vi "AndorSnap.vi"() -> ()   [LabVIEW 2014]
uses:
  <userlib>/atmcd64d.llb/AcquisitionMode_mode typedef.ctl
  <userlib>/atmcd64d.llb/ReadMode_mode typedef.ctl
  <userlib>/atmcd64d.llb/Shutter_mode typedef.ctl
  <userlib>/atmcd64d.llb/Shutter_type typedef.ctl
  <userlib>/atmcd64d.llb/TriggerMode_mode typedef.ctl
  <userlib>/atmcd64d.llb/Error Code Enum typedef.ctl
panel:
  out "SaveStatus":bool
  in  "FilePath":string="C:\\Users\\light\\Desktop\\Chuanzhen\\Andor\\data"
  out "ShutDown":cluster{"CoolOff":bool, "ShutDown":bool}
  in  "Set":bool
  in  "Snap":bool
  out "SetStatus":bool
  out "SetOut":T1
  out "Timing":T2 {"kinetic" format="%.2f"; "accumulate" format="%.2f"; "exposure" format="%.2f"}
  in  "MultiTrack":cluster{"StartRow":i32, "EndRow":i32}={"StartRow"=1, "EndRow"=256}
  in  "AcqSet":T3={"openingtime"=20, "closingtime"=20, "ExposureTime"=0.01, "AccumCycTime"=0.0, "AccumCycNum"=1, "KineticNum"=1, "KineticTime"=0.0} {"KineticTime" format="%.2f"; "AccumCycTime" format="%.2f"; "ExposureTime" format="%.2f"}
  in  "Mode":T9={"AcqMode"=enum."Single Scan", "ReadMode"=enum."Image", "ShutterMode"=enum."Auto", "GateMode"=enum."TTL High", "TriggerMode"=enum."Internal"}
  in  "Exit":bool
  out "CoolerON":T10
  out "CurrentTemp":i32
  out "GetStatus":T11
  out "Speeds":T12
  out "SoftWVersion":T13
  out "HardWVersion":T14
  out "DevSize":cluster{"xpixels":i32, "ypixels":i32}
  out "DevInit":bool
  in  "TargetTemp":i32
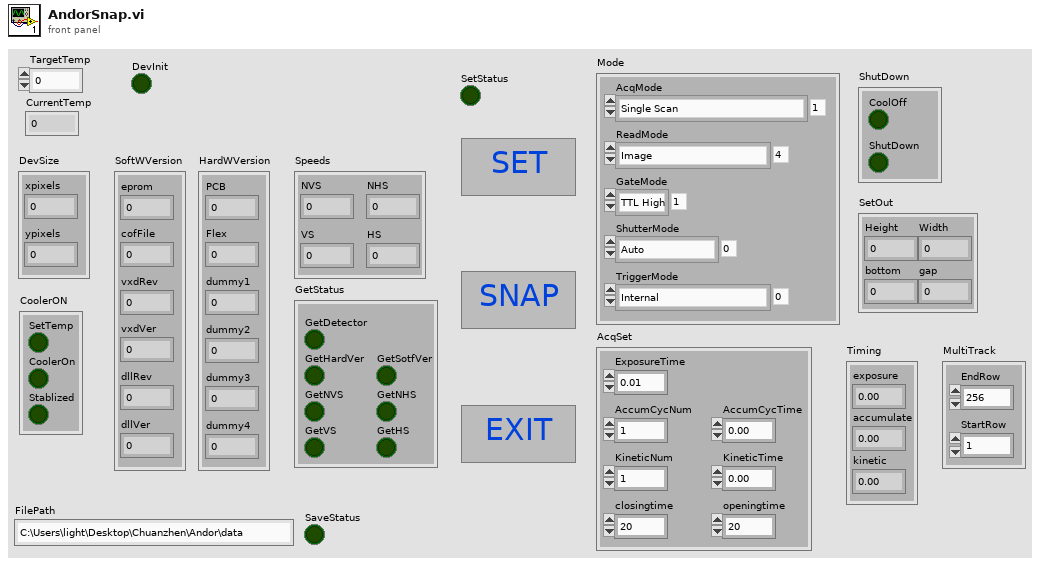
[diagram p1: front panel]
types:
  T1 = cluster{"Height":i32, "Width":i32, "bottom":i32, "gap":i32}
  T2 = cluster{"exposure":sgl, "accumulate":sgl, "kinetic":sgl}
  T3 = cluster{"openingtime":i32, "closingtime":i32, "ExposureTime":sgl, "AccumCycTime":sgl, "AccumCycNum":i32, "KineticNum":i32, "KineticTime":sgl}
  T4 = typedef "AcquisitionMode_mode typedef.ctl" = enum16{"Reserved (0)", "Single Scan", "Accumulate", "Kinetics", "Fast Kinetics", "Run Till Abort", "Reserved (6)", "Reserved (7)", "Reserved (8)", "Time Delayed Integration"}
  T5 = typedef "ReadMode_mode typedef.ctl" = enum16{"Full Vertical Binning", "Multi-Track", "Random-Track", "Single-Track", "Image"}
  T6 = typedef "Shutter_mode typedef.ctl" = enum16{"Auto", "Open", "Close", "N/A (3)", "Open FVB Series", "Open Any Series"}
  T7 = typedef "Shutter_type typedef.ctl" = enum16{"TTL Low", "TTL High"}
  T8 = typedef "TriggerMode_mode typedef.ctl" = enum16{"Internal", "External", "N/A (2)", "N/A (3)", "N/A (4)", "N/A (5)", "External Start", "External Exposure (Bulb)", "N/A (8)", "External FVB EM", "Software", "N/A (11)", "External Charge Shifting"}
  T9 = cluster{"AcqMode":T4, "ReadMode":T5, "ShutterMode":T6, "GateMode":T7, "TriggerMode":T8}
  T10 = cluster{"SetTemp":bool, "CoolerOn":bool, "Stablized":bool}
  T11 = cluster{"GetDetector":bool, "GetHardVer":bool, "GetNVS":bool, "GetVS":bool, "GetSotfVer":bool, "GetNHS":bool, "GetHS":bool}
  T12 = cluster{"NVS":i32, "VS":i32, "NHS":dbl, "HS":i32}
  T13 = cluster{"eprom":u32, "cofFile":u32, "vxdRev":u32, "vxdVer":u32, "dllRev":u32, "dllVer":u32}
  T14 = cluster{"PCB":u32, "Flex":u32, "dummy1":u32, "dummy2":u32, "dummy3":u32, "dummy4":u32}
  T15 = typedef "Error Code Enum typedef.ctl" = enum32{"N/A (0)", "DRV_ERROR_CODES", "DRV_SUCCESS", "DRV_VXDNOTINSTALLED", "DRV_ERROR_SCAN", "DRV_ERROR_CHECK_SUM", "DRV_ERROR_FILELOAD", "DRV_UNKNOWN_FUNC", "DRV_ERROR_VXD_INIT", "DRV_ERROR_ADDRESS", "DRV_ERROR_PAGELOCK", "DRV_ERROR_PAGEUNLOCK", "DRV_ERROR_BOARDTEST", "DRV_ERROR_ACK", "DRV_ERROR_UP_FIFO", "DRV_ERROR_PATTERN", "N/A (16)", "DRV_ACQUISITION_ERRORS", "DRV_ACQ_BUFFER", "DRV_ACQ_DOWNFIFO_FULL", "DRV_PROC_UNKONWN_INSTRUCTION", "DRV_ILLEGAL_OP_CODE", "DRV_KINETIC_TIME_NOT_MET", "DRV_ACCUM_TIME_NOT_MET", "DRV_NO_NEW_DATA", "N/A (25)", "DRV_SPOOLERROR", "N/A (27)", "N/A (28)", "N/A (29)", "N/A (30)", "N/A (31)", "N/A (32)", "DRV_TEMPERATURE_CODES", "DRV_TEMPERATURE_OFF", "DRV_TEMPERATURE_NOT_STABILIZED", "DRV_TEMPERATURE_STABILIZED", "DRV_TEMPERATURE_NOT_REACHED", "DRV_TEMPERATURE_OUT_RANGE", "DRV_TEMPERATURE_NOT_SUPPORTED", "DRV_TEMPERATURE_DRIFT", "N/A (41)", "N/A (42)", "N/A (43)", "N/A (44)", "N/A (45)", "N/A (46)", "N/A (47)", "N/A (48)", "DRV_GENERAL_ERRORS", "DRV_INVALID_AUX", "DRV_COF_NOTLOADED", "DRV_FPGAPROG", "DRV_FLEXERROR", "DRV_GPIBERROR", "N/A (55)", "N/A (56)", "N/A (57)", "N/A (58)", "N/A (59)", "N/A (60)", "N/A (61)", "N/A (62)", "N/A (63)", "DRV_DATATYPE", "DRV_DRIVER_ERRORS", "DRV_P1INVALID", "DRV_P2INVALID", "DRV_P3INVALID", "DRV_P4INVALID", "DRV_INIERROR", "DRV_COFERROR", "DRV_ACQUIRING", "DRV_IDLE", "DRV_TEMPCYCLE", "DRV_NOT_INITIALIZED", "DRV_P5INVALID", "DRV_P6INVALID", "DRV_INVALID_MODE", "DRV_INVALID_FILTER", "DRV_I2CERRORS", "DRV_I2CDEVNOTFOUND", "DRV_I2CTIMEOUT", "DRV_P7INVALID", "N/A (84)", "N/A (85)", "N/A (86)", "N/A (87)", "N/A (88)", "N/A (89)", "DRV_IOCERROR", "DRV_VRMVERSIONERROR"}
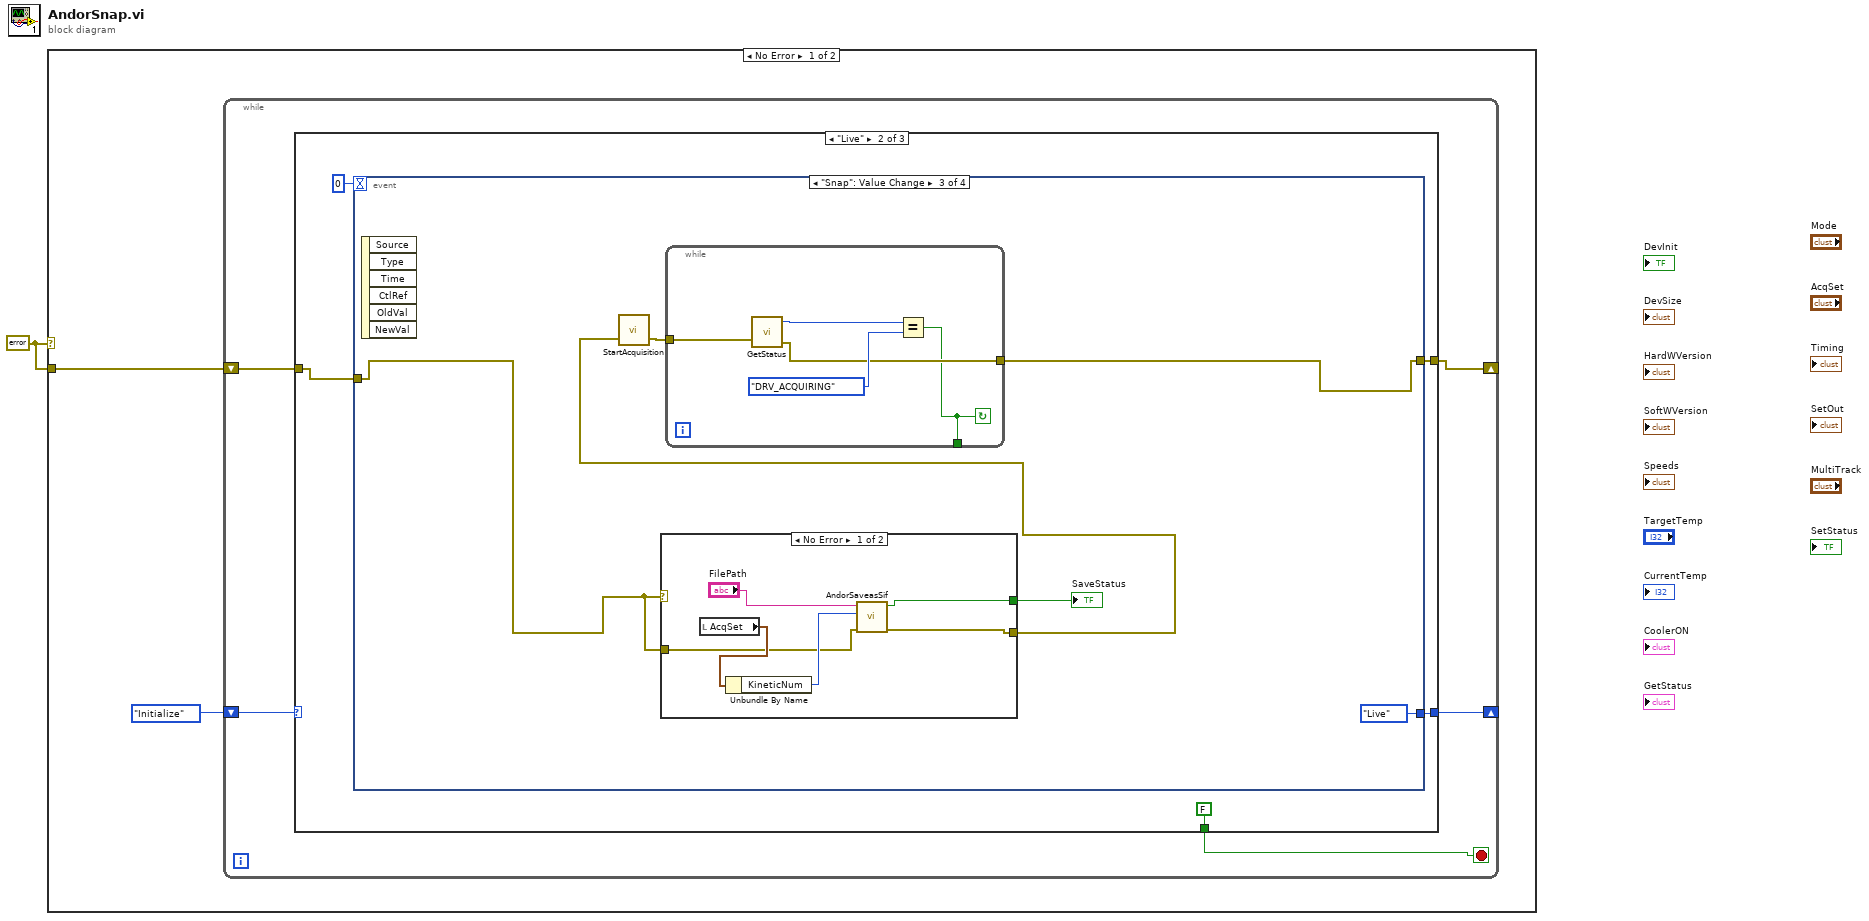
[diagram p0: block diagram]
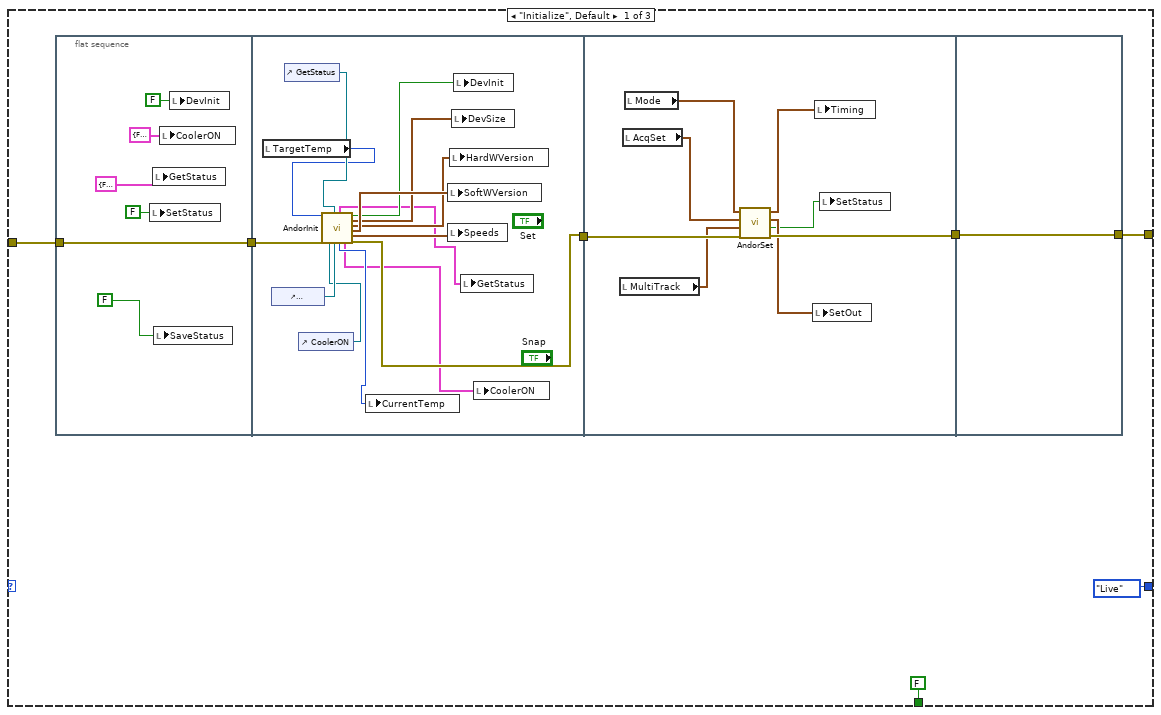
[diagram p2: hidden frame]
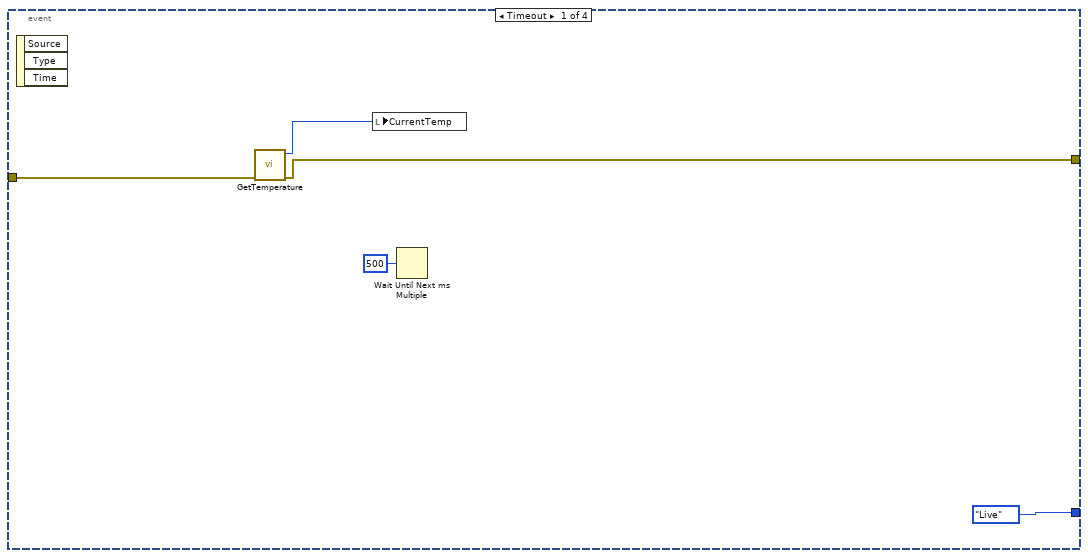
[diagram p3: hidden frame]
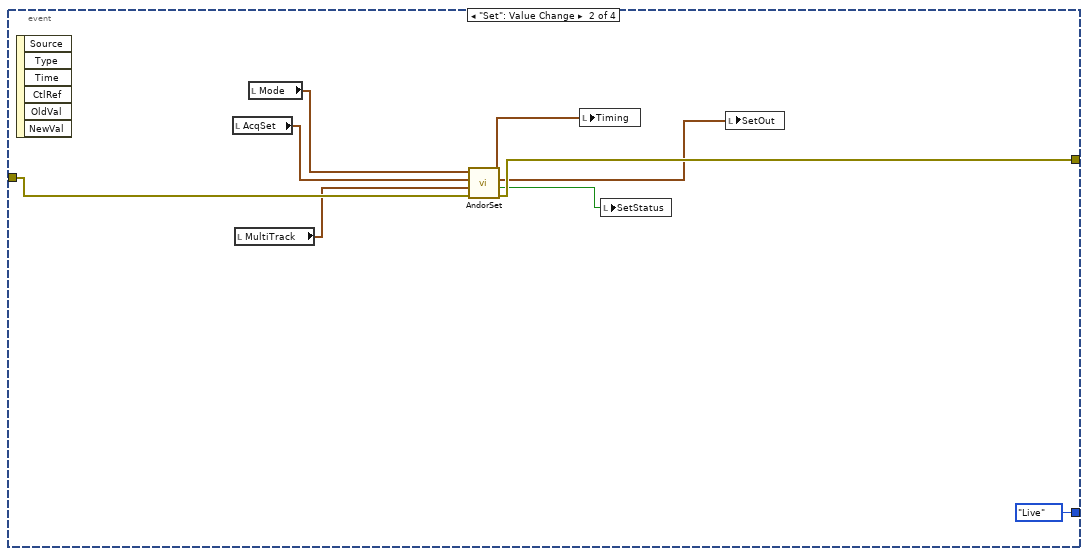
[diagram p4: hidden frame]
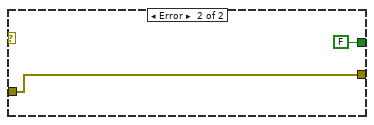
[diagram p5: hidden frame]
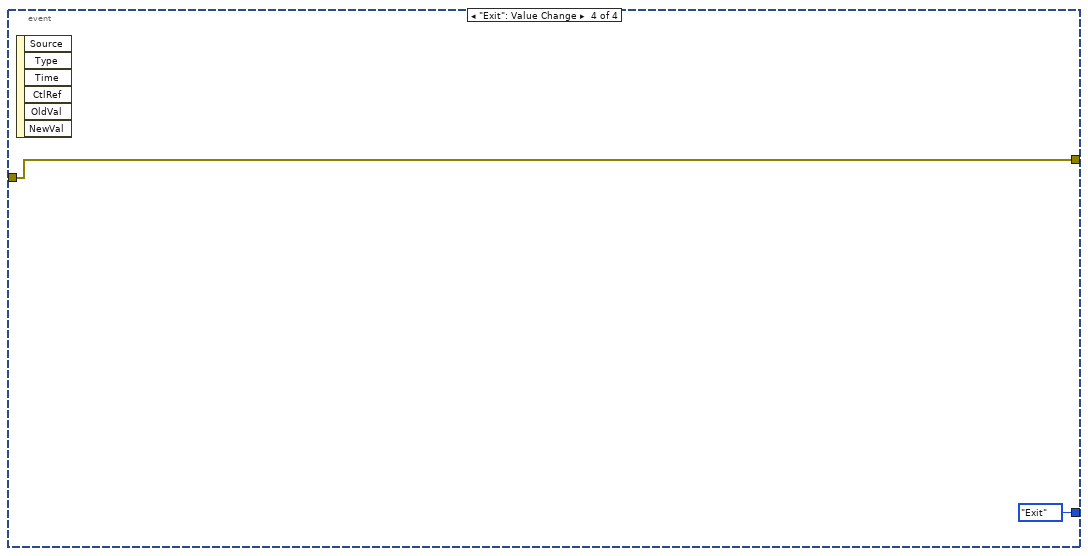
[diagram p6: hidden frame]
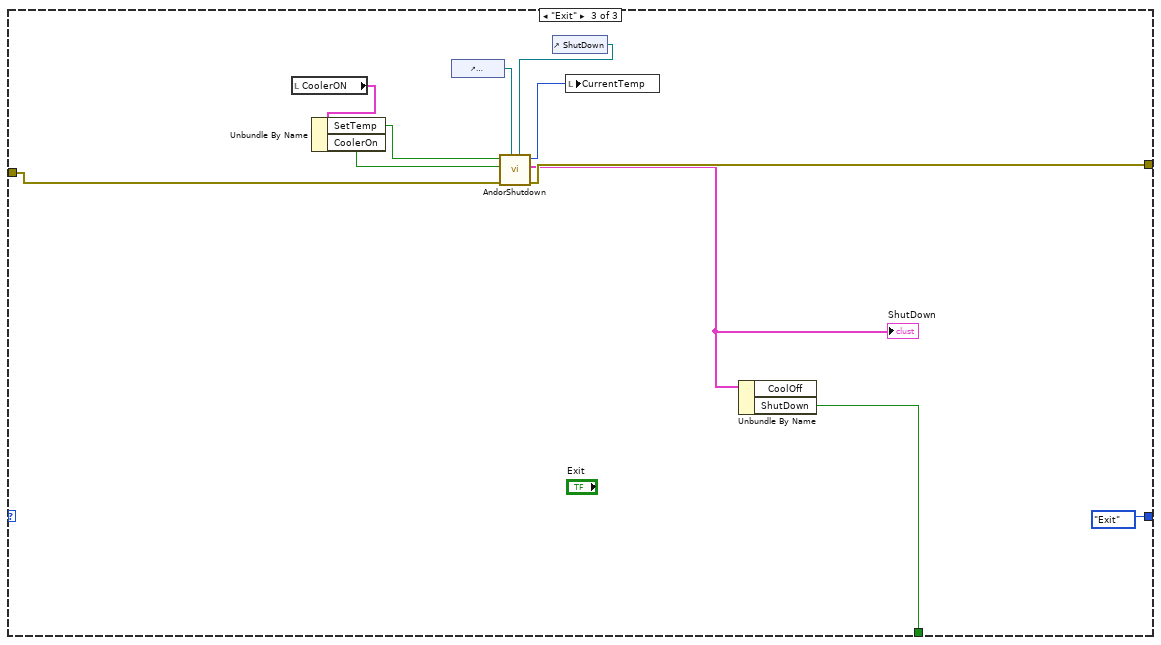
[diagram p7: hidden frame]
diagram:
  w1 = errorcluster {"status"=FALSE, "code"=0, "source"=""} ("error in")
  n1 = case shown="No Error" w1 {
    tunnel: w1 -> [w2 _]
    frame No Error {
      n2 = while {
        shift-right: [w7] -> _
        shift-left: enum16{"Initialize", "Live", "Exit"}."Initialize" -> [w8]
        shift-right: [w5] -> _
        shift-left: w2 -> [w6]
        stop <- w4 stop-if-true
        n3 = case shown="\"Live\"" w8 {
          tunnel: [enum16{"Initialize", "Live", "Exit"}."Live" w49 enum16{"Initialize", "Live", "Exit"}."Exit"] -> w7
          tunnel: w6 -> [w13 w48 w94]
          tunnel: [w10 w47 w93] -> w5
          tunnel: [FALSE ("ShutDown") FALSE ("ShutDown") w85] -> w4
          frame "Initialize", Default {
            n4 = flat-sequence {
              tunnel: [w21] -> w14
              tunnel: w13 -> [w21]
              tunnel: w14 -> [w35]
              tunnel: [w34] -> w12
              tunnel: w12 -> [w43]
              tunnel: [w42] -> w11
              tunnel: w11 -> [w44]
              tunnel: [w44] -> w10
              frame #0 {
                n5 = local write "SetStatus"(FALSE ("SetStatus")) -> ()
                n6 = local write "GetStatus"(T11 {"GetDetector"=FALSE, "GetHardVer"=FALSE, "GetNVS"=FALSE, "GetVS"=FALSE, "GetSotfVer"=FALSE, "GetNHS"=FALSE, "GetHS"=FALSE} ("GetStatus")) -> ()
                n7 = local write "SaveStatus"(FALSE ("Save")) -> ()
                n8 = local write "CoolerON"(T10 {"SetTemp"=FALSE, "CoolerOn"=FALSE, "Stablized"=FALSE} ("CoolerON")) -> ()
                n9 = local write "DevInit"(FALSE ("DevInit")) -> ()
              }
              frame #1 {
                n10 = local read "TargetTemp"() -> (w30:i32)
                n11 = control-ref of="CurrentTemp"() -> (w32:refnum<vi>)
                n12 = control-ref of="GetStatus"() -> (w33:refnum<vi>)
                n13 = control-ref of="CoolerON"() -> (w31:refnum<vi>)
                n14 = call "AndorInit.vi"("TargetTemp"=w30, "error in"=w35, "CoolerONRef"=w31, "GetStatusRef"=w33, "CurrentTempRef"=w32) -> ("GetStatus"=w22:T11, "CurrentTemp"=w29:i32, "CoolerON"=w28:T10, "DevInit"=w25:bool, "DevSize"=w24:cluster{"xpixels":i32, "ypixels":i32}, "HardWVersion"=w23:T14, "SoftWVersion"=w26:T13, "Speeds"=w27:T12, "error out"=w34:errorcluster)  [unwired: 6 in]
                n15 = local write "CurrentTemp"(w29) -> ()
                n16 = local write "SoftWVersion"(w26) -> ()
                n17 = local write "Speeds"(w27) -> ()
                n18 = local write "HardWVersion"(w23) -> ()
                n19 = local write "DevSize"(w24) -> ()
                n20 = local write "DevInit"(w25) -> ()
                n21 = local write "GetStatus"(w22) -> ()
                n22 = local write "CoolerON"(w28) -> ()
              }
              frame #2 {
                n23 = local read "MultiTrack"() -> (w39:cluster{"StartRow":i32, "EndRow":i32})
                n24 = local read "AcqSet"() -> (w41:T3)
                n25 = local read "Mode"() -> (w40:T9)
                n26 = call "AndorSet.vi"("error in"=w43, "MultiTrack"=w39, "AcqSet"=w41, "Mode"=w40) -> ("error out"=w42:errorcluster, "SetStatus"=w36:bool, "SetOut"=w37:T1, "Timing"=w38:T2)  [unwired: 4 in]
                n27 = local write "SetOut"(w37) -> ()
                n28 = local write "Timing"(w38) -> ()
                n29 = local write "SetStatus"(w36) -> ()
              }
              frame #3 {
              }
            }
          }
          frame "Live" {
            n30 = event shown="[2] \"Snap\": Value Change" {
              selector: _ -> [_ _ _ _]
              dyn-events: _ -> [_ _ _ _]
              timeout: 0 -> [_ _ _ _]
              tunnel: [enum16{"Initialize", "Live", "Exit"}."Live" enum16{"Initialize", "Live", "Exit"}."Live" enum16{"Initialize", "Live", "Exit"}."Live" enum16{"Initialize", "Live", "Exit"}."Exit"] -> w49
              tunnel: w48 -> [w51 w62 w66 w83]
              tunnel: [w50 w61 w64 w83] -> w47
              event Timeout {
                n31 = event-data() -> ()  [unwired: 1 in, 3 out]
                n32 = call <userlib>:"GetTemperature.vi"("error in (no error)"=w51) -> ("error out"=w50:errorcluster, "temperature"=w53:i32)  [unwired: 3 in, 2 out]
                n33 = local write "CurrentTemp"(w53) -> ()
                n34 = Wait Until Next ms Multiple(millisecond multiple=u32 500) -> ()  [unwired: 1 out]
              }
              event "Set": Value Change {
                n35 = event-data() -> ()  [unwired: 1 in, 6 out]
                n36 = local read "AcqSet"() -> (w59:T3)
                n37 = local read "MultiTrack"() -> (w58:cluster{"StartRow":i32, "EndRow":i32})
                n38 = local read "Mode"() -> (w60:T9)
                n39 = call "AndorSet.vi"("error in"=w62, "MultiTrack"=w58, "AcqSet"=w59, "Mode"=w60) -> ("error out"=w61:errorcluster, "SetStatus"=w56:bool, "SetOut"=w55:T1, "Timing"=w57:T2)  [unwired: 4 in]
                n40 = local write "Timing"(w57) -> ()
                n41 = local write "SetStatus"(w56) -> ()
                n42 = local write "SetOut"(w55) -> ()
              }
              event "Snap": Value Change {
                n43 = event-data() -> ()  [unwired: 1 in, 6 out]
                n44 = case shown="No Error" w66 {
                  tunnel: w66 -> [w72 w77]
                  tunnel: [w70 FALSE ("SaveStatus")] -> w67
                  tunnel: [w71 w77] -> w65
                  frame No Error {
                    n45 = local read "AcqSet"() -> (w74:T3)
                    n46 = Unbundle By Name(w74) -> ("KineticNum"=w73:i32)
                    n47 = call "AndorSaveasSif.vi"("error in"=w72, "KinNumber"=w73, "FilePath"="FilePath") -> ("error out"=w71:errorcluster, "SaveStatus"=w70:bool)  [unwired: 7 in]
                  }
                  frame Error {
                  }
                }
                "SaveStatus" <- w67
                n48 = call <userlib>:"StartAcquisition.vi"("error in (no error)"=w65) -> ("error out"=w68:errorcluster)  [unwired: 1 in, 1 out]
                n49 = while {
                  tunnel: w68 -> [w82]
                  tunnel: [w79] -> w64
                  tunnel: [w78] -> _
                  stop <- w78 continue-if-true
                  n50 = call <userlib>:"GetStatus.vi"("error in (no error)"=w82) -> ("error out"=w79:errorcluster, "status"=w81:T15)  [unwired: 2 in, 1 out]
                  n51 = Equal?(x=w81, y=Error_Code_Enum_typedef."DRV_ACQUIRING") -> (x = y?=w78:bool)
                }
              }
              event "Exit": Value Change {
                n52 = event-data() -> ()  [unwired: 1 in, 6 out]
              }
            }
          }
          frame "Exit" {
            n53 = local read "CoolerON"() -> (w92:T10)
            n54 = Unbundle By Name(w92) -> ("SetTemp"=w91:bool, "CoolerOn"=w90:bool)
            n55 = control-ref of="CurrentTemp"() -> (w89:refnum<vi>)
            n56 = control-ref of="ShutDown"() -> (w87:refnum<vi>)
            n57 = call "AndorShutdown.vi"("ShutDownRef"=w87, "CurrentTempRef"=w89, "error in"=w94, "CoolerON"=w90, "SetTemp"=w91) -> ("error out"=w93:errorcluster, "ShutDown"=w86:cluster{"CoolOff":bool, "ShutDown":bool}, "CurrentTemp"=w88:i32)  [unwired: 4 in]
            "ShutDown" <- w86
            n58 = local write "CurrentTemp"(w88) -> ()
            n59 = Unbundle By Name(w86) -> ("ShutDown"=w85:bool)  [unwired: 1 out]
          }
        }
      }
    }
    frame Error {
    }
  }
